vi "Keysight_N6700C_TurnOn.vi"(6 "error in (no error)":errorcluster {"code" format="%.0x"}, 7 "VISA resource name":refnum<visa-resource-name>, 8 "Current_CH2":dbl=2.0 format="%#_13g", 9 "Voltage_CH2":dbl=12.0 format="%#_13g", 10 "Current_CH1":dbl=6.0 format="%#_13g", 11 "Voltage_CH1":dbl=12.0) -> (0 "error out":errorcluster {"code" format="%.0x"}, 3 "VISA resource name out":refnum<visa-resource-name>)   [LabVIEW 2018]
doc: "Turn On Power Supply\nChannel 1: 12V, 8A\nChannel 2: 12V, 2A"
uses:
  SupportVIs/Agilent N6700 Series.lvlib
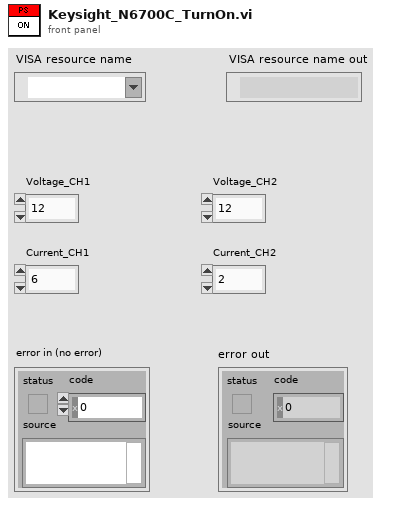
[diagram p1: front panel]
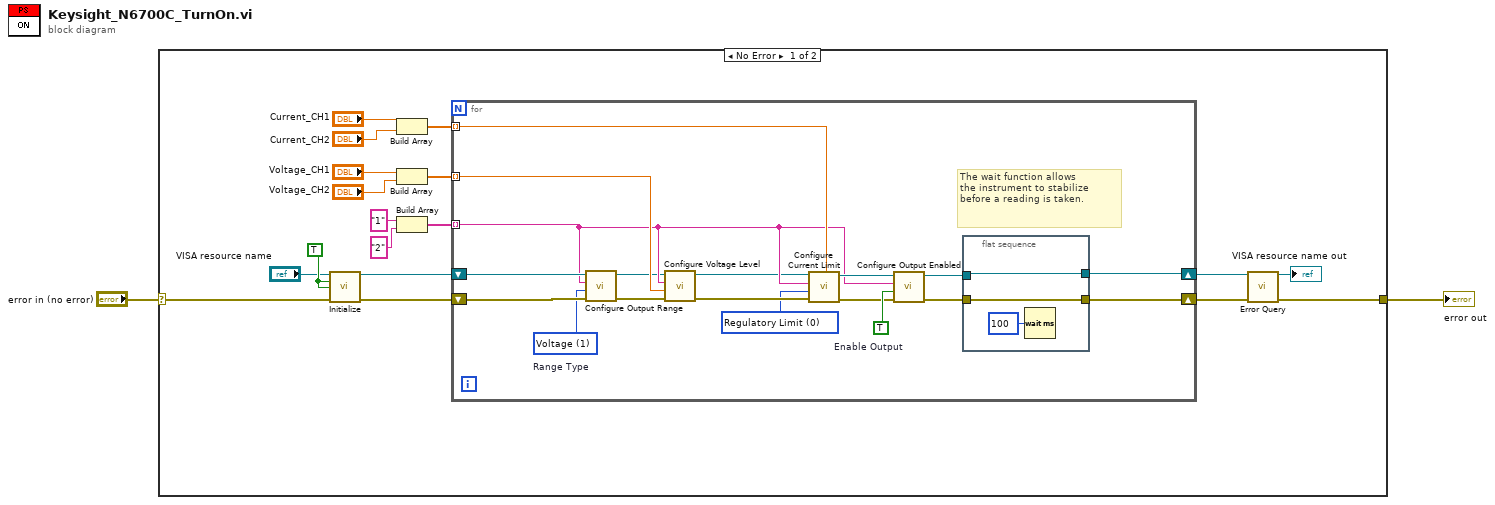
[diagram p0: block diagram]
diagram:
  n1 = case shown="No Error" "error in (no error)" {
    selector: "error in (no error)" -> [w3 w42]
    tunnel: [w9 w42] -> w2
    frame No Error {
      w7 = TRUE ("Reset? (T: Yes)")
      n2 = call "Initialize.vi"("VISA resource name"="VISA resource name", "ID Query? (T: Yes)"=w7, "Reset? (T: Yes)"=w7, "error in (no error)"=w3) -> ("VISA resource name out"=w5:refnum<visa-resource-name>, "error out"=w4:errorcluster)  [unwired: 10 in]
      n3 = Build Array("Current_CH1", "Current_CH2") -> (w15:dbl[])
      n4 = Build Array("Voltage_CH1", "Voltage_CH2") -> (w14:dbl[])
      n5 = Build Array("1" ("Channel Name (1)"), "2" ("Channel Name (2)")) -> (w13:string[])
      n6 = for {
        tunnel: w15 -> [w35] mode=indexing
        tunnel: w14 -> [w28] mode=indexing
        tunnel: w13 -> [w27] mode=indexing
        shift-right: [w33] -> w19
        shift-left: w5 -> [w30]
        shift-right: [w32] -> w20
        shift-left: w4 -> [w29]
        w21 = 0 items=["Regulatory Limit", "Trip Limit"] ("Behavior (0: Regulatory Limit)")
        w24 = 1 items=["Voltage"=1, "Current"=0]  # Range Type
        w38 = TRUE  # Enable Output
        # "The wait function allows \nthe instrument to stabilize\nbefore a reading is taken."
        n7 = call "Configure Output Range.vi"("error in (no error)"=w29, "Range Type (1: Voltage)"=w24, "Channel Name (1)"=w27, "VISA resource name"=w30) -> ("error out"=w23:errorcluster, "VISA resource name out"=w22:refnum<visa-resource-name>)  [unwired: 6 in]
        n8 = call "Configure Voltage Level.vi"("error in (no error)"=w23, "Level  (0.0 volts)"=w28, "Channel Name (1)"=w27, "VISA resource name"=w22) -> ("error out"=w26:errorcluster, "VISA resource name out"=w25:refnum<visa-resource-name>)  [unwired: 6 in]
        n9 = call "Configure Current Limit.vi"("Limit (0.0 amps)"=w35, "error in (no error)"=w26, "Behavior (0: Regulatory Limit)"=w21, "Channel Name (1)"=w27, "VISA resource name"=w25) -> ("error out"=w37:errorcluster, "VISA resource name out"=w36:refnum<visa-resource-name>)  [unwired: 5 in]
        n10 = call "Configure Output Enabled.vi"("error in (no error)"=w37, "Enable Output (False)"=w38, "Channel Name (1)"=w27, "VISA resource name"=w36) -> ("error out"=w31:errorcluster, "VISA resource name out"=w34:refnum<visa-resource-name>)  [unwired: 6 in]
        n11 = flat-sequence {
          tunnel: w34 -> [w41]
          tunnel: [w41] -> w33
          tunnel: [w39] -> w32
          tunnel: w31 -> [w39]
          frame #0 {
            n12 = Wait (ms)(milliseconds to wait=u32 100) -> ()  [unwired: 1 out]
          }
        }
      }
      n13 = call "Error Query.vi"("VISA resource name"=w19, "error in (no error)"=w20) -> ("VISA resource name out"=→"VISA resource name out":refnum<visa-resource-name>, "error out"=w9:errorcluster)  [unwired: 10 in, 2 out]
    }
    frame Error {
    }
  }
  "error out" <- w2
